vi "PH_SSAC.PC Set Frame.vi"(0 "i ref in":refnum<vi>, 2 "Signal":T1, 3 "Frame":cluster{"x":u32, "dx":u32, "y":u32, "dy":u32}, 5 "error IO":errorcluster) -> (14 "i ref out":refnum<vi>, 19 "error out":errorcluster)   [LabVIEW 2014, in "PH_SSAC.lvlib"]
uses:
  PH_SSAC.lvlib
  PH_SSAC.Signal Selector.ctl
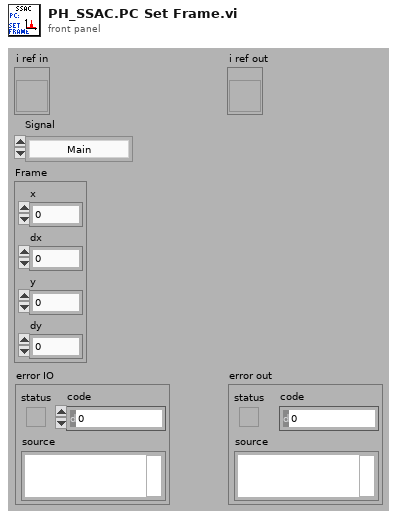
[diagram p1: front panel]
types:
  T1 = typedef "PH_SSAC.lvlib/PH_SSAC.Signal Selector.ctl" = enum16{"Main", "Background"}
  T2 = typedef "PH_SSAC.lvlib/PH_SSAC.i attribute.ctl" = cluster{"GUI Refs":cluster{"Delete":refnum<vi>, "Global On":refnum<vi>, "Cam Source":refnum<vi>, "Frame Main Signal":refnum<vi>, "Frame Background":refnum<vi>, "dt (Gauss smooth)":refnum<vi>, "Calibration Factor":refnum<vi>, "Background acquire":refnum<vi>, "Threshold":refnum<vi>, "Time evolution of mean pulse duration":refnum<vi>, "Mean Pulse Duration":refnum<vi>, "Main signal":refnum<vi>, "Current Pulse Duration":refnum<vi>, "Processed":refnum<vi>, "Saturation":refnum<vi>, "# for Average":refnum<vi>, "Position":refnum<vi>, "BG Status":refnum<vi>, "Save BG data":refnum<vi>, "Read BG Data":refnum<vi>, "Background Calibration Data":refnum<vi>}, "Images":cluster{"OP Image":T3, "GUI Image":T3, "PSDB Image":T3}, "Global On?":bool, "Frame Main":cluster{"x":u32, "dx":u32, "y":u32, "dy":u32}, "Frame Background":cluster{"x":u32, "dx":u32, "y":u32, "dy":u32}, "dt [fs]":dbl, "Calibration Factor [fs/pixel]":dbl, "Threshold":dbl, "Time evolution of mean pulse duration [fs]":dbl[], "Main Signal":cluster{"Time for Main":dbl[], "Signal":dbl[]}, "Processed":bool, "Current Pulse Duration [fs]":dbl, "# for Average":i32, "Position":i32, "Pulse Durations [fs]":dbl[], "BG":cluster{"Acquire?":bool, "Background Calibration Data":T4, "Save Data":bool}}
  T3 = typedef "IMAQ Image.ctl" = refnum<image>
  T4 = typedef "PH_SSAC.lvlib/PH_SSAC.Background Data.ctl" = cluster{"Date":string, "Time":string, "Frame Main":cluster{"x":u32, "dx":u32, "y":u32, "dy":u32}, "dt [fs]":dbl, "Calibration Factor [fs/pixel]":dbl, "Signal":dbl[], "Frame Background":cluster{"x":u32, "dx":u32, "y":u32, "dy":u32}}
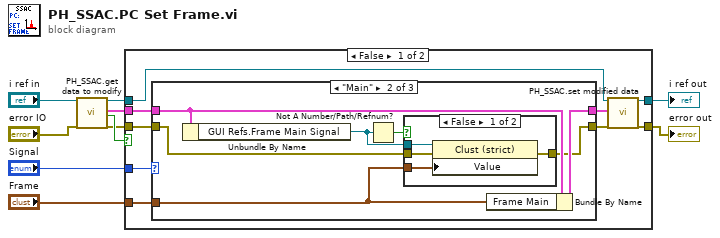
[diagram p0: block diagram]
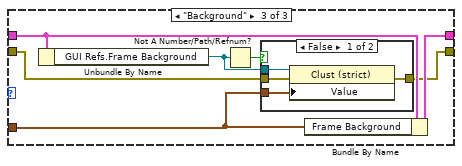
[diagram p4: hidden frame]
diagram:
  n1 = call "PH_SSAC.get data to modify.vi"("i ref in"="i ref in", "error in (no error)"="error IO") -> ("i ref out"=w4:refnum<vi>, "i attribute"=w10:T2, "timed out"=w9:bool, "error out"=w3:errorcluster)  [unwired: 14 in]
  n2 = case shown="False" w9 {
    tunnel: w3 -> [w15 w46]
    tunnel: w4 -> [w11 w47]
    tunnel: [w19 w47] -> w6
    tunnel: [w18 w46] -> w8
    tunnel: w10 -> [w16 _]
    tunnel: "Frame" -> [w13 _]
    tunnel: "Signal" -> [w12 _]
    frame False {
      n3 = case shown="\"Main\"" w12 {
        tunnel: [w21 w28 w40] -> w17
        tunnel: w16 -> [w21 w27 w39]
        tunnel: w15 -> [w20 w26 w38]
        tunnel: [w20 w25 w37] -> w14
        tunnel: w13 -> [_ w24 w36]
        frame Default {
        }
        frame "Main" {
          n4 = Unbundle By Name(w27) -> ("GUI Refs.Frame Main Signal"=w22:refnum<vi>)
          n5 = Not A Number/Path/Refnum?(number/path/refnum=w22) -> (NaN/Path/Refnum?=w23:bool)
          n6 = case shown="False" w23 {
            tunnel: w26 -> [w32 w33]
            tunnel: [w31 w33] -> w25
            tunnel: w22 -> [w30 _]
            tunnel: w24 -> [w29 _]
            frame False {
              n7 = property class="Clust (strict)"(reference=w30, error in=w32, "Value"=w29) -> (error out=w31:errorcluster)  [unwired: 1 out]
            }
            frame True {
            }
          }
          n8 = Bundle By Name(cluster=w27, "Frame Main"=w24) -> (w28:T2)
        }
        frame "Background" {
          n9 = Unbundle By Name(w39) -> ("GUI Refs.Frame Background"=w34:refnum<vi>)
          n10 = Not A Number/Path/Refnum?(number/path/refnum=w34) -> (NaN/Path/Refnum?=w35:bool)
          n11 = case shown="False" w35 {
            tunnel: w38 -> [w44 w45]
            tunnel: [w43 w45] -> w37
            tunnel: w34 -> [w42 _]
            tunnel: w36 -> [w41 _]
            frame False {
              n12 = property class="Clust (strict)"(reference=w42, error in=w44, "Value"=w41) -> (error out=w43:errorcluster)  [unwired: 1 out]
            }
            frame True {
            }
          }
          n13 = Bundle By Name(cluster=w39, "Frame Background"=w36) -> (w40:T2)
        }
      }
      n14 = call "PH_SSAC.set modified data.vi"("i ref in"=w11, "i attribute"=w17, "error in (no error)"=w14) -> ("i ref out"=w19:refnum<vi>, "error out"=w18:errorcluster)  [unwired: 15 in]
    }
    frame True {
    }
  }
  "error out" <- w8
  "i ref out" <- w6
